vi "Operator message space bar continue.vi"(8 "error in (no error)":errorcluster, 10 "Message.Font:Size":u32=36, 11 "Message":string) -> (0 "error out":errorcluster, 3 "Time waiting in secs":string)   [LabVIEW 2013]
uses:
  <vilib>/event_ctls.llb/eventvkey.ctl
panel:
  # "Operator Message"
  # "Press SPACE BAR to continue"
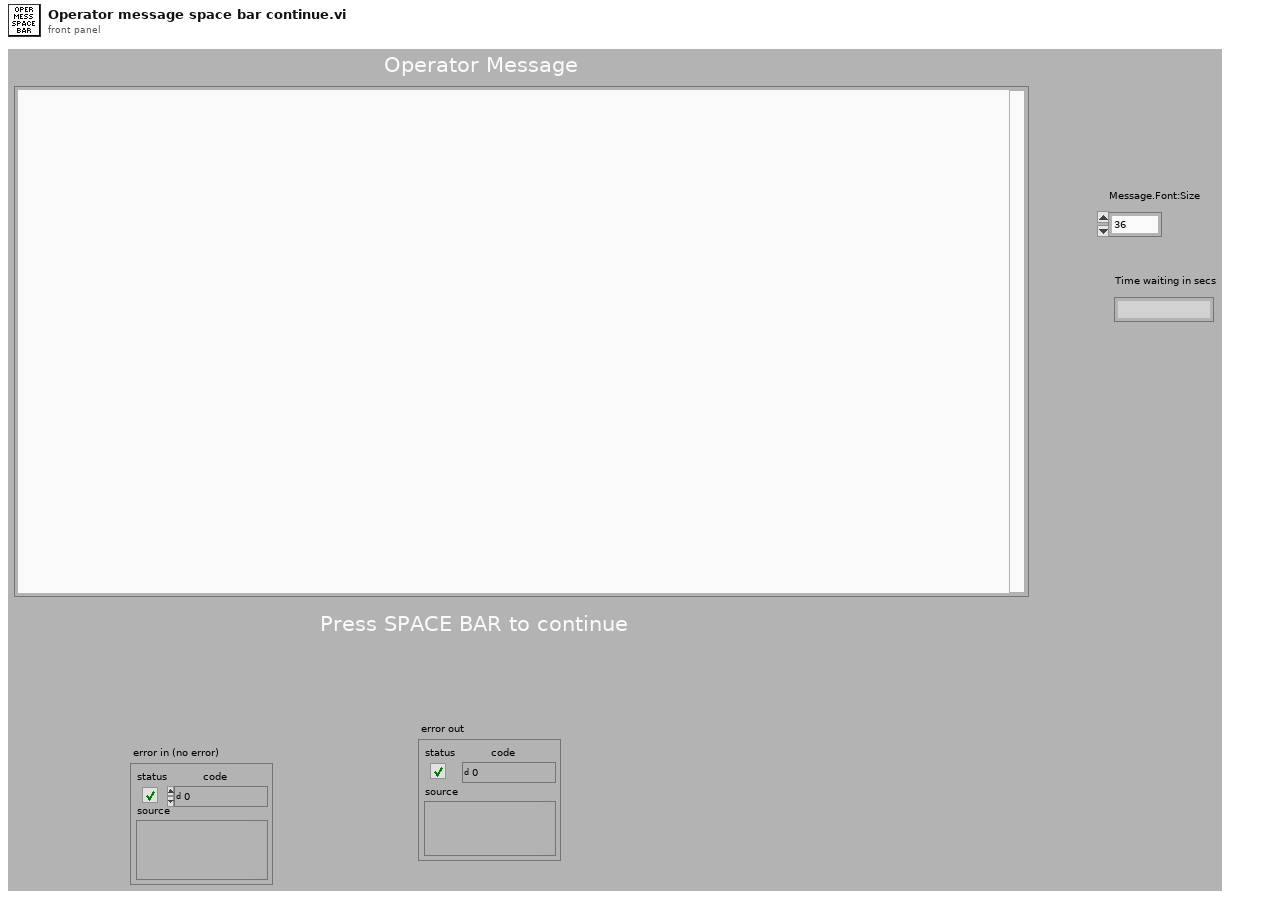
[diagram p1: front panel]
types:
  T1 = typedef "eventvkey.ctl" = enum16{"ASCII", "Enter", "Return", "Shift", "Ctrl", "Alt", "Cmd", "Opt", "Caps", "NumLock", "Clear", "Break", "Up", "Down", "Left", "Right", "Insert", "Delete", "Home", "End", "PageUp", "PageDown", "Escape", "Help", "Pause", "ScrollLock", "F1", "F2", "F3", "F4", "F5", "F6", "F7", "F8", "F9", "F10", "F11", "F12", "F13", "F14", "F15", "F16", "F17", "F18", "F19", "F20", "F21", "F22", "F23", "F24", "Play", "VolumeUp", "VolumeDown", "Mute", "Two Byte Char"}
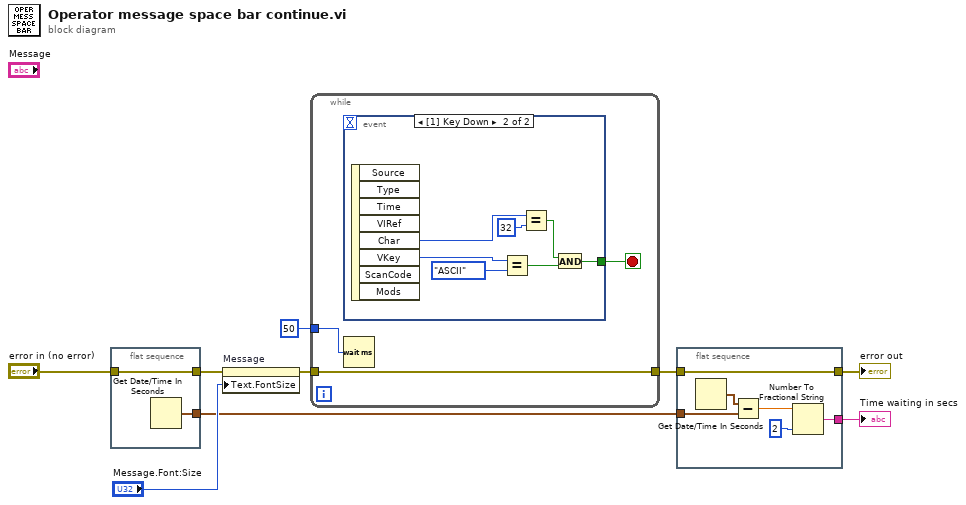
[diagram p0: block diagram]
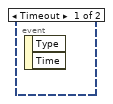
[diagram p2: hidden frame]
diagram:
  n1 = flat-sequence {
    tunnel: [w11] -> w6
    tunnel: "error in (no error)" -> [w11]
    tunnel: [w10] -> w2
    frame #0 {
      n2 = Get Date/Time In Seconds() -> (seconds since 1Jan1904=w10:timestamp)
    }
  }
  n3 = property on="Message" class="Str"(error in=w6, "Text.FontSize"="Message.Font:Size") -> (error out=w8:errorcluster)  [unwired: 1 in, 1 out]
  n4 = while {
    tunnel: u32 50 ("milliseconds to wait") -> [w14]
    tunnel: [w12] -> w4
    tunnel: w8 -> [w12]
    stop <- w13 stop-if-true
    n5 = event shown="[1] Key Down" {
      selector: _ -> [_ _]
      dyn-events: _ -> [_ _]
      timeout: _ -> [_ _]
      tunnel: [_ w15] -> w13
      event Timeout {
        n6 = event-data() -> ()  [unwired: 1 in, 2 out]
      }
      event Key Down {
        n7 = event-data() -> ("Char"=w21:i16, "VKey"=w19:T1)  [unwired: 1 in, 6 out]
        n8 = Equal?(x=w19, y=eventvkey."ASCII" ("VKey")) -> (x = y?=w16:bool)
        n9 = Equal?(x=w21, y=i16 32) -> (x = y?=w17:bool)
        n10 = And(x=w17, y=w16) -> (x .and. y?=w15:bool)
      }
    }
    n11 = Wait (ms)(milliseconds to wait=w14) -> ()  [unwired: 1 out]
  }
  n12 = flat-sequence {
    tunnel: [w27] -> w3
    tunnel: w4 -> [w27]
    tunnel: w2 -> [w25]
    tunnel: [w22] -> w1
    frame #0 {
      n13 = Get Date/Time In Seconds() -> (seconds since 1Jan1904=w26:timestamp)
      n14 = Subtract(x=w26, y=w25) -> (x-y=w24:dbl)
      n15 = Number To Fractional String(number=w24, precision (6)=i16 2) -> (F-format string=w22:string)  [unwired: 2 in]
    }
  }
  "error out" <- w3
  "Time waiting in secs" <- w1
